vi "ex1-3.vi"() -> ()   [LabVIEW 2019]
panel:
  in  "stop":bool
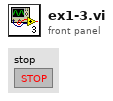
[diagram p1: front panel]
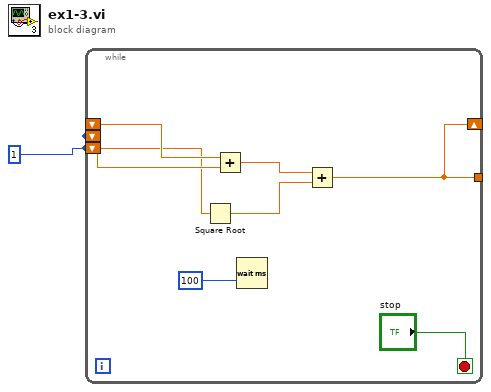
[diagram p0: block diagram]
diagram:
  w1 = 1
  n1 = while {
    shift-right: [w3] -> _
    shift-left: w1 -> [w9]
    shift-left: w1 -> [w8]
    shift-left: w1 -> [w7]
    tunnel: [w3] -> _
    stop <- "stop" stop-if-true
    n2 = Square Root(x=w7) -> (sqrt(x)=w6:dbl)
    n3 = Add(x=w9, y=w8) -> (x+y=w5:dbl)
    n4 = Wait (ms)(milliseconds to wait=100) -> ()  [unwired: 1 out]
    n5 = Add(x=w5, y=w6) -> (x+y=w3:dbl)
  }
